vi "Initialize.vi"(8 "error in (no error)":errorcluster, 11 "FunctionGenerator in":refnum<class "FunctionGenerator.lvclass">) -> (0 "error out":errorcluster, 3 "FunctionGenerator out":refnum<class "FunctionGenerator.lvclass">)   [LabVIEW 2020, in "FunctionGenerator.lvclass"]
doc: "VIRTUAL FUNCTION\n\nThis VI should be overwritten by methods using the specific initialization procedure for the respective child class."
uses:
  FunctionGenerator.lvclass
  C:/Code Projects/CircuitExplorer/AnalogDiscoveryFunction/AnalogDiscoveryFunction.lvclass
  AnalogDiscoveryFunction/AnalogDiscoveryFunction.lvclass/AnalogDiscoveryFunction.ctl
  AnalogDiscoveryFunction/GetDeviceName.vi
  AnalogDiscoveryFunction/SetInstrumentHandle.vi
  <vilib>/DigilentWF/DigilentWF.lvlib
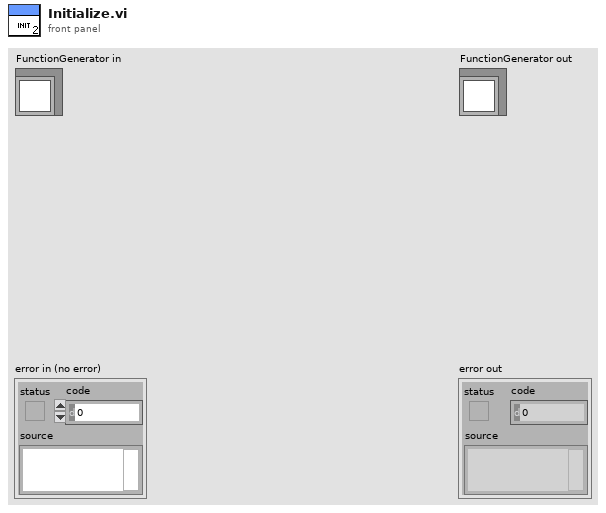
[diagram p1: front panel]
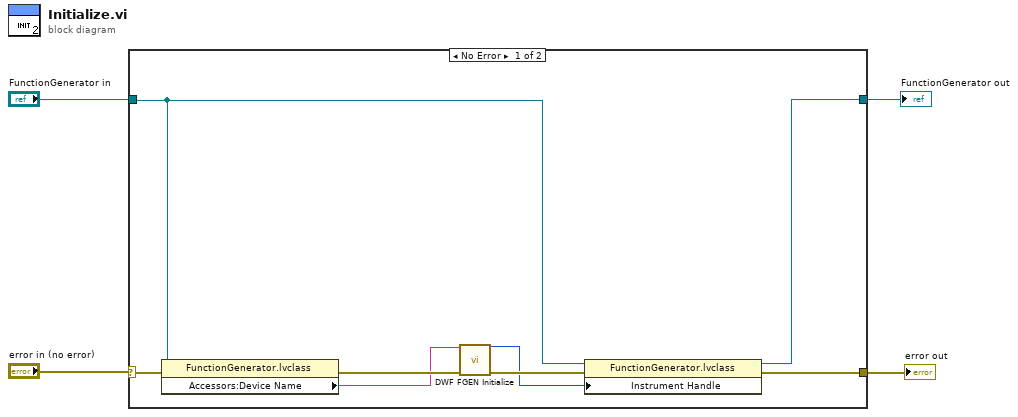
[diagram p0: block diagram]
diagram:
  n1 = case shown="No Error" "error in (no error)" {
    selector: "error in (no error)" -> [w12 w14]
    tunnel: [w8 w14] -> w3
    tunnel: "FunctionGenerator in" -> [w6 w13]
    tunnel: [w5 w13] -> w1
    frame No Error {
      n2 = property class="FunctionGenerator.lvclass"(reference=w6, error in=w12) -> (error out=w11:errorcluster, "Accessors:Device Name"=w10:string)  [unwired: 1 out]
      n3 = call <vilib>:"DWF FGEN Initialize.vi"("Device Name"=w10, "Error In"=w11) -> ("Instrument Handle Out"=w7:u32, "Error Out"=w9:errorcluster)  [unwired: 12 in]
      n4 = property class="FunctionGenerator.lvclass"(reference=w6, error in=w9, "Instrument Handle"=w7) -> (reference out=w5:refnum<class "FunctionGenerator.lvclass">, error out=w8:errorcluster)
    }
    frame Error {
    }
  }
  "error out" <- w3
  "FunctionGenerator out" <- w1
